vi "OPENUSB.vi"() -> (1 "N DISPOSITIVOS":i32, 2 "PIPE OUT":i32, 3 "PIPE in":i32)   [LabVIEW 2016]
uses:
  mpusbapi.dll
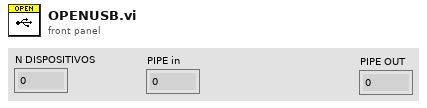
[diagram p1: front panel]
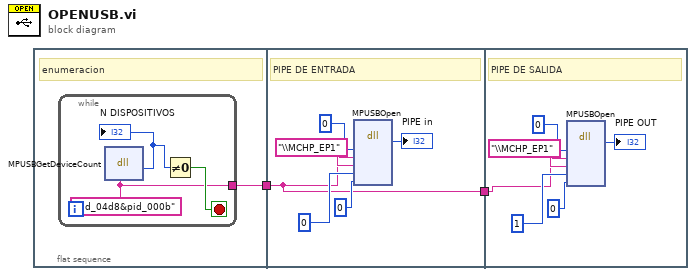
[diagram p0: block diagram]
diagram:
  n1 = flat-sequence {
    tunnel: [w3] -> w2
    tunnel: w2 -> [w7]
    tunnel: [w7] -> w1
    tunnel: w1 -> [w13]
    frame #0 {
      # "enumeracion"
      n2 = while {
        tunnel: [w4] -> w3
        stop <- w5 stop-if-true
        w4 = "vid_04d8&pid_000b" ("pVID_PID")
        n3 = dll-call lib="mpusbapi.dll" fn="MPUSBGetDeviceCount"("pVID_PID"=w4) -> ("N DISPOSITIVOS"=w6:i32)  [unwired: 4 in, 2 out]
        "N DISPOSITIVOS" <- w6
        n4 = Not Equal To 0?(x=w6) -> (x != 0?=w5:bool)
      }
    }
    frame #1 {
      # "PIPE DE ENTRADA"
      n5 = dll-call lib="mpusbapi.dll" fn="MPUSBOpen"("INSTNCIA"=0, "PID_VID"=w7, "pEP"="\\MCHP_EP1", "dwDIR"=0, "dwReserved"=0) -> ("PIPE"=→"PIPE in":i32)  [unwired: 8 in, 2 out]
    }
    frame #2 {
      # "PIPE DE SALIDA"
      n6 = dll-call lib="mpusbapi.dll" fn="MPUSBOpen"("INSTNCIA"=0, "PID_VID"=w13, "pEP"="\\MCHP_EP1", "dwDIR"=1, "dwReserved"=0) -> ("PIPE"=→"PIPE OUT":i32)  [unwired: 8 in, 2 out]
    }
  }
